vi "Read 1Chan NSamp Waveform.vi"(8 "error in (no error)":errorcluster, 9 "timeout [s]":dbl=-1.0, 10 "number of samples per channel":i32=1000, 11 "MicroDAQ.lvlib:Analog Input.lvclass":refnum<class "Analog Input.lvclass">) -> (0 "error out":errorcluster, 2 "Values":waveform(dbl), 3 "MicroDAQ.lvlib:Analog Input.lvclass out":refnum<class "Analog Input.lvclass">)   [LabVIEW 2009, in "MicroDAQ.lvlib" / "Analog Input.lvclass"]
doc: "Reads a waveform from a channel."
uses:
  <instrlib>/MicroDAQ/Channel/Analog Input/Analog Input.lvclass
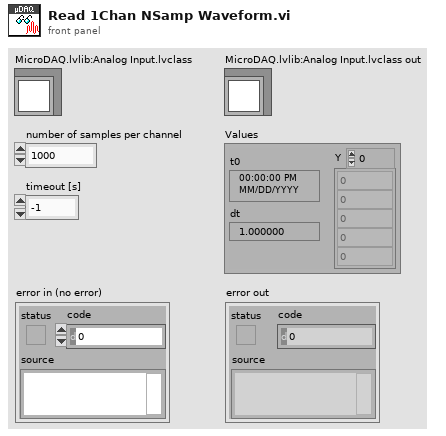
[diagram p1: front panel]
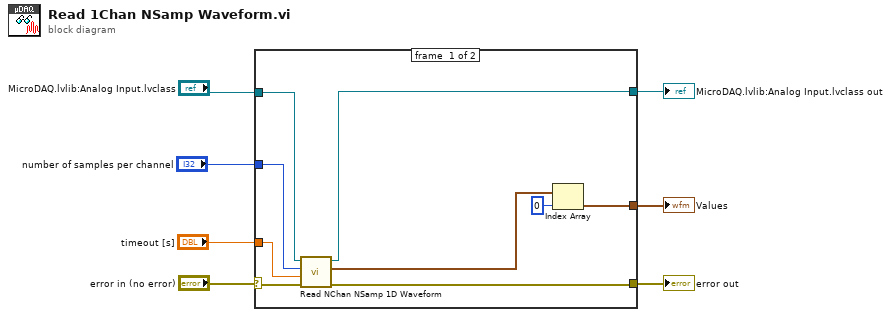
[diagram p0: block diagram]
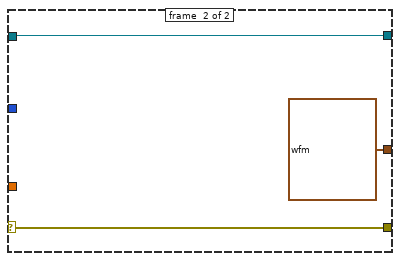
[diagram p2: hidden frame]
diagram:
  n1 = case shown="No Error" "error in (no error)" {
    selector: "error in (no error)" -> [w16 w18]
    tunnel: [w12 w18] -> w6
    tunnel: [w13 w19] -> w5
    tunnel: "number of samples per channel" -> [w14 _]
    tunnel: "MicroDAQ.lvlib:Analog Input.lvclass" -> [w15 w19]
    tunnel: [w9 waveform(dbl) {"t0"=timestamp(0 s since 1904-01-01), "dt"=1.0, "Y"=[]} ("Waveform")] -> w2
    tunnel: "timeout [s]" -> [w8 _]
    frame #0 {
      n2 = call <instrlib>:"Read NChan NSamp 1D Waveform.vi"("error in (no error)"=w16, "timeout [s]"=w8, "number of samples per channel"=w14, "MicroDAQ.lvlib:Analog Input.lvclass"=w15) -> ("error out"=w12:errorcluster, "Values"=w10:waveform(dbl)[], "MicroDAQ.lvlib:Analog Input.lvclass out"=w13:refnum<class "Analog Input.lvclass">)  [unwired: 5 in]
      n3 = Index Array(array=w10, index=0) -> (element=w9:waveform(dbl))
    }
    frame #1 {
    }
  }
  "error out" <- w6
  "MicroDAQ.lvlib:Analog Input.lvclass out" <- w5
  "Values" <- w2
